vi "image processing (SubVI).vi"(2 "error in":errorcluster, 3 "Image dst":T1, 4 "Image src":T1) -> (0 "error out":errorcluster, 1 "Image Out":T1)   [LabVIEW 2009]
uses:
  <vilib>/vision/Image Controls.llb/IMAQ Image.ctl
  <vilib>/vision/NI_Vision_Development_Module.lvlib
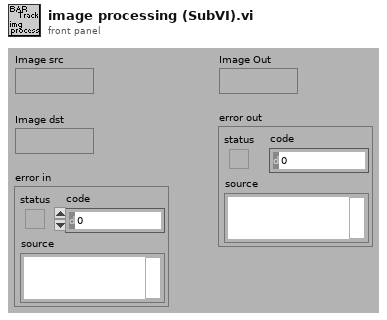
[diagram p1: front panel]
types:
  T1 = typedef "IMAQ Image.ctl" = refnum<image>
  T2 = enum32{"AutoM", "Close", "Dilate", "Erode", "Gradient", "Gradient in", "Gradient out", "HitMiss", "Open", "PClose", "POpen", "Thick", "Thin"}
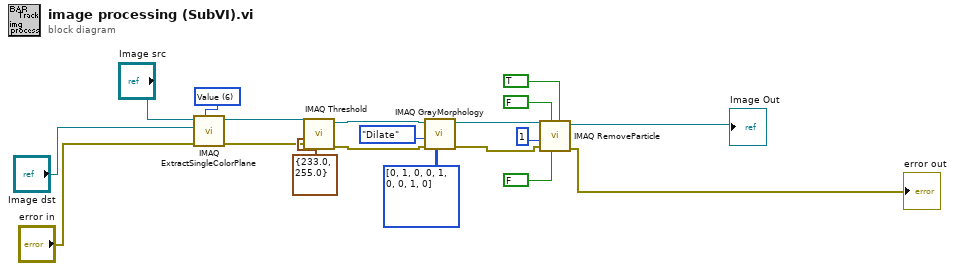
[diagram p0: block diagram]
diagram:
  w1 = 6 items=["Red", "Green", "Blue", "Hue", "Saturation", "Luminance", "Value", "Intensity"] ("Color Plane")
  n1 = call "IMAQ ExtractSingleColorPlane"("Color Plane"=w1, "error in (no error)"="error in", "Image Dst"="Image dst", "Image Src"="Image src") -> ("error out"=w2:errorcluster, "Image Dst Out"=w3:T1)  [unwired: 6 in]
  n2 = call "IMAQ Threshold"("error in (no error)"=w2, "Range"=cluster{"Lower value":sgl, "Upper value":sgl} {"Lower value"=233.0, "Upper value"=255.0}, "Image Src"=w3) -> ("error out"=w4:errorcluster, "Image Dst Out"=w7:T1)  [unwired: 7 in]
  n3 = call "IMAQ GrayMorphology"("Structuring Element"=i32[][] [[0, 1, 0], [0, 1, 0], [0, 1, 0]], "error in (no error)"=w4, "Operation"=T2."Dilate", "Image Src"=w7) -> ("error out"=w8:errorcluster, "Image Dst Out"=w13:T1)  [unwired: 6 in]
  n4 = call "IMAQ RemoveParticle"("Connectivity 4/8 (8)"=TRUE, "Low Pass/High Pass (Low)"=FALSE, "Square/Hexa (Square)"=FALSE, "error in (no error)"=w8, "Number of Erosion"=1, "Image Src"=w13) -> ("error out"=→"error out":errorcluster, "Image Dst Out"=→"Image Out":T1)  [unwired: 4 in]
